vi "Adv_GetXMLFromLightField.vi"(8 "error in (no error)":errorcluster, 10 "Path In":path, 11 "LightField Automation in":refnum<class "LightField Automation.lvclass">) -> (0 "error out":errorcluster, 1 "XML FNS":string, 2 "XML FDS":string, 3 "LightField Automation out":refnum<class "LightField Automation.lvclass">)   [LabVIEW 2015, in "LightField Automation.lvclass"]
uses:
  LightField Automation.lvclass
  LightField Automation.lvclass/LightField Automation.ctl
  C:/Program Files/Princeton Instruments/LightField/AddInViews/PrincetonInstruments.LightFieldViewV3.dll
  Program Files/Princeton Instruments/LightField/AddInViews/PrincetonInstruments.LightFieldViewV3.dll
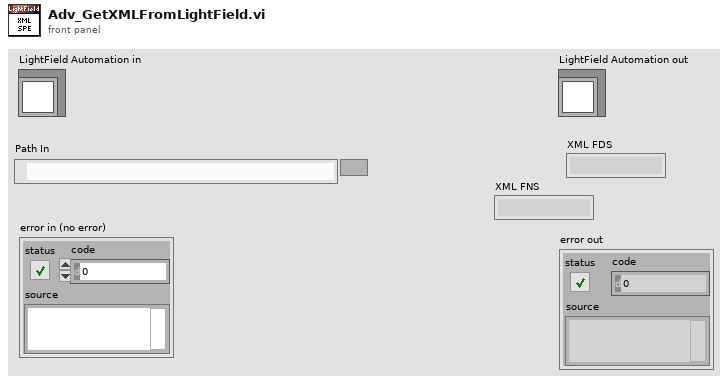
[diagram p1: front panel]
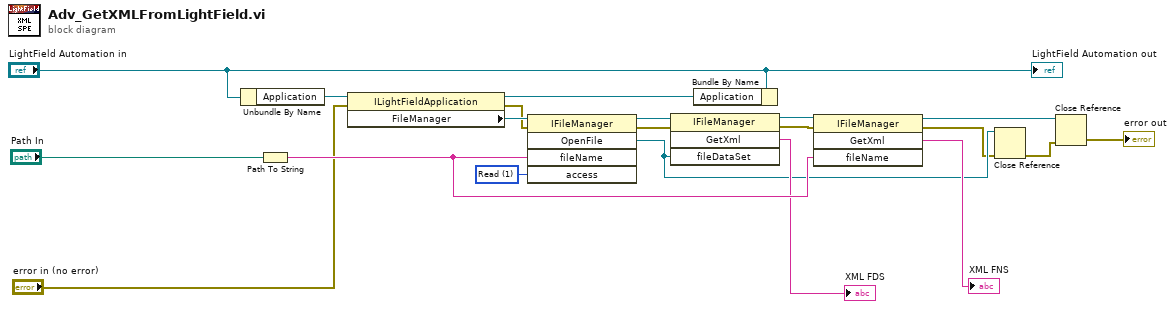
[diagram p0: block diagram]
diagram:
  w17 = 1 items=["Read"=1, "Write"=2, "ReadWrite"=3] ("access")
  n1 = Unbundle By Name("LightField Automation in") -> ("Application"=w20:refnum<k24>)
  n2 = Path To String(path="Path In") -> (string=w14:string)
  n3 = property class="ILightFieldApplication"(reference=w20, error in="error in (no error)") -> (reference out=w11:refnum<k24>, error out=w3:errorcluster, "FileManager"=w19:refnum<k24>)
  n4 = invoke class="IFileManager" method="OpenFile"(reference=w19, error in=w3, "fileName"=w14, "access"=w17) -> (reference out=w16:refnum<k24>, error out=w4:errorcluster, "OpenFile"=w9:refnum<k24>)  [unwired: 1 in, 2 out]
  n5 = invoke class="IFileManager" method="GetXml"(reference=w16, error in=w4, "fileDataSet"=w9) -> (reference out=w15:refnum<k24>, error out=w5:errorcluster, "GetXml"=→"XML FDS":string)  [unwired: 1 in, 1 out]
  n6 = Bundle By Name(cluster="LightField Automation in", "Application"=w11) -> ()  [unwired: 1 out]
  n7 = invoke class="IFileManager" method="GetXml"(reference=w15, error in=w5, "fileName"=w14) -> (reference out=w8:refnum<k24>, error out=w7:errorcluster, "GetXml"=→"XML FNS":string)  [unwired: 1 in, 1 out]
  n8 = Close Reference(reference=w9, error in (no error)=w7) -> (error out=w6:errorcluster)
  n9 = Close Reference(reference=w8, error in (no error)=w6) -> (error out=→"error out":errorcluster)
  "LightField Automation out" <- "LightField Automation in"
